vi "FindReachableVertices.vi"(5 "source":i32, 9 "DAG in":refnum<class "DAG.lvclass">) -> (4 "reachable":bool[](array[boolean]))   [LabVIEW 2014, in "DAG.lvclass"]
uses:
  DAG.lvclass
  DAG.lvclass/DAG.ctl
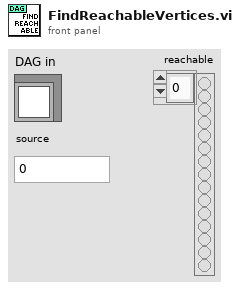
[diagram p1: front panel]
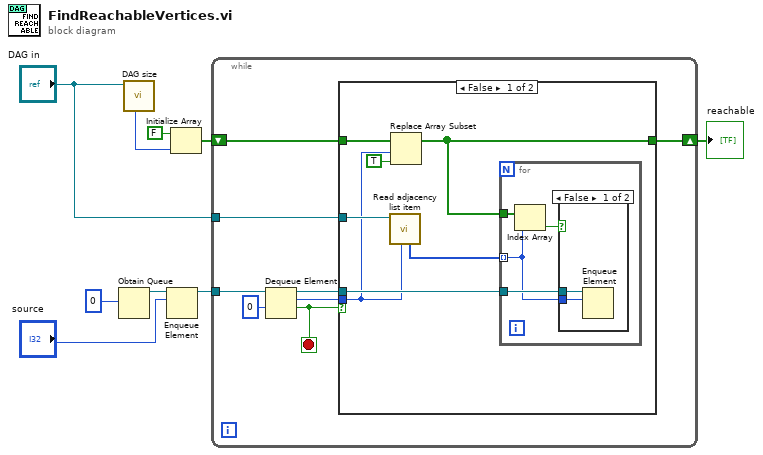
[diagram p0: block diagram]
diagram:
  n1 = Obtain Queue(element data type=0) -> (queue out=w6:refnum<queue>)  [unwired: 4 in, 2 out]
  n2 = call "DAG size.vi"("DAG in"="DAG in") -> ("vertices"=w8:i32)  [unwired: 6 in, 2 out]
  n3 = Enqueue Element(queue=w6, element="source") -> (queue out=w5:refnum<queue>)  [unwired: 2 in, 2 out]
  n4 = Initialize Array(FALSE, w8) -> (w3:bool[])
  n5 = while {
    shift-right: [w13] -> w4
    shift-left: w3 -> [w12]
    tunnel: w5 -> [w17]
    tunnel: "DAG in" -> [w10]
    stop <- w14 stop-if-true
    n6 = Dequeue Element(queue=w17, timeout in ms (-1)=0) -> (queue out=w15:refnum<queue>, element=w11:i32, timed out?=w14:bool)  [unwired: 1 in, 1 out]
    n7 = case shown="False" w14 {
      tunnel: w15 -> [w22 _]
      tunnel: [w19 w31] -> w13
      tunnel: w12 -> [w24 w31]
      tunnel: w11 -> [w20 _]
      tunnel: w10 -> [w21 _]
      frame False {
        n8 = call "Read adjacency list item.vi"("vertex"=w20, "DAG in"=w21) -> ("edge list"=w18:i32[])  [unwired: 6 in, 1 out]
        n9 = Replace Array Subset(array=w24, new element=TRUE ("new element/subarray"), index=w20) -> (w19:bool[])
        n10 = for {
          tunnel: w18 -> [w26] mode=indexing
          tunnel: w22 -> [w28]
          tunnel: w19 -> [w27]
          n11 = Index Array(array=w27, index=w26) -> (element=w25:bool)
          n12 = case shown="False" w25 {
            tunnel: w28 -> [w30 _]
            tunnel: w26 -> [w29 _]
            frame False {
              n13 = Enqueue Element(queue=w30, element=w29) -> ()  [unwired: 2 in, 3 out]
            }
            frame True {
            }
          }
        }
      }
      frame True {
      }
    }
  }
  "reachable" <- w4
